vi "Modbus LDO Sensors.vi"(8 "error in":errorcluster, 11 "PLC Data":T1) -> (0 "error out":errorcluster, 3 "PLC Data Output":T1)   [LabVIEW 2020, in "Modbus.lvlib"]
uses:
  Modbus.lvlib
  Modbus PLC Data All.ctl
  Modbus FVIR Control.ctl
  Modbus LDO Control.ctl
  WritingDataFile/Data to Save.ctl
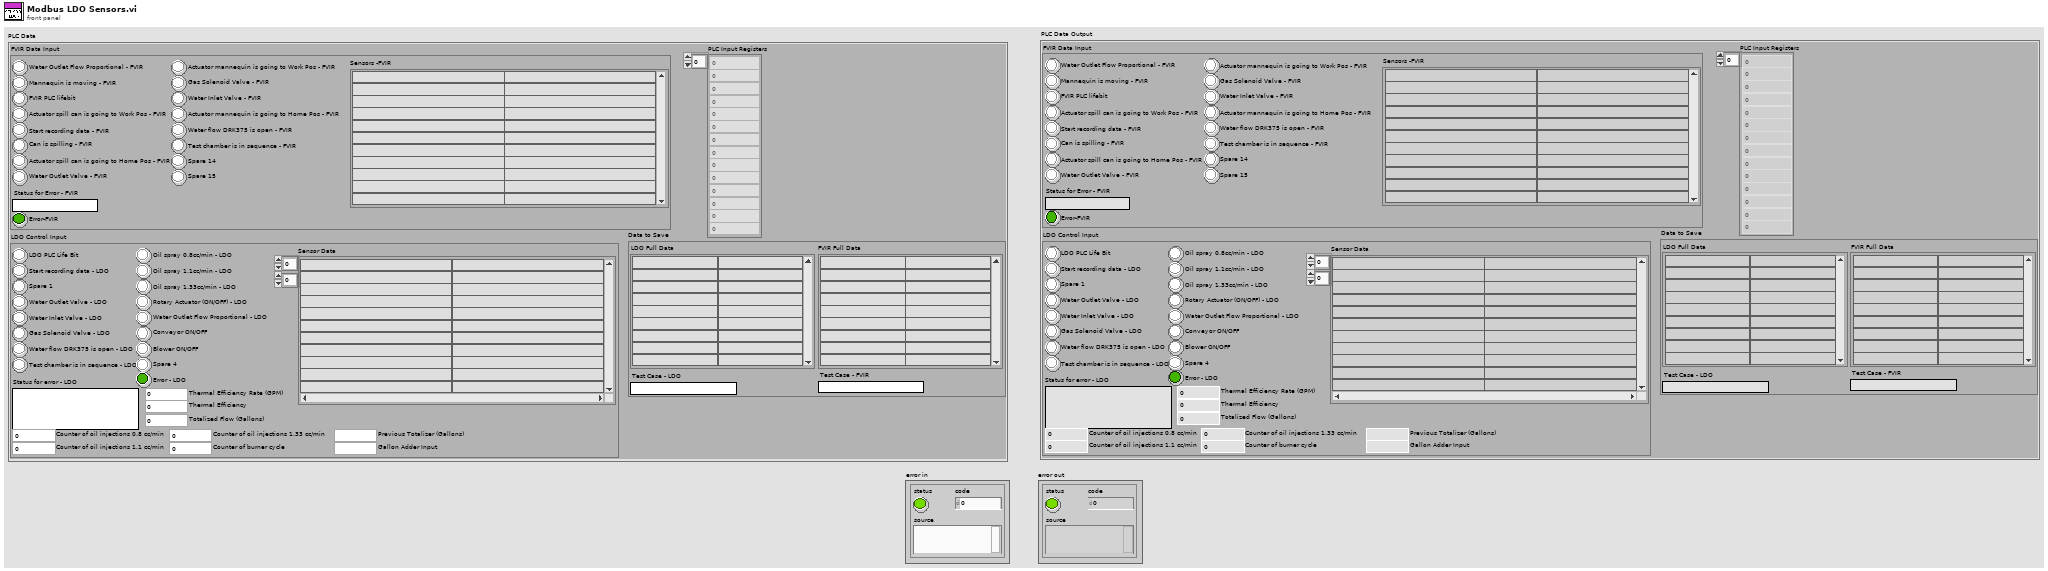
[diagram p1: front panel]
types:
  T1 = typedef "Modbus PLC Data All.ctl" = cluster{"FVIR Data Input":T2, "LDO Control Input":T3, "PLC Input Registers":i16[], "Data to Save":T4}
  T2 = typedef "Modbus FVIR Control.ctl" = cluster{"Spare 15":bool, "Spare 14":bool, "Actuator mannequin is going to Work Pos - FVIR":bool, "Actuator mannequin is going to Home Pos - FVIR":bool, "Test chamber is in sequence - FVIR ":bool, "Water flow DRK375 is open - FVIR":bool, "Gas Solenoid Valve - FVIR":bool, "Water Inlet Valve - FVIR":bool, "Water Outlet Flow Proportional - FVIR":bool, "Start recording data - FVIR":bool, "Actuator spill can is going to Work Pos - FVIR":bool, "Actuator spill can is going to Home Pos - FVIR":bool, "Water Outlet Valve - FVIR":bool, "Can is spilling - FVIR":bool, "Mannequin is moving - FVIR":bool, "FVIR PLC lifebit":bool, "Status for Error - FVIR":string, "Error-FVIR":bool, "Sensors -FVIR":string[][]}
  T3 = typedef "Modbus LDO Control.ctl" = cluster{"LDO PLC Life Bit":bool, "Start recording data - LDO":bool, "Spare 1":bool, "Water Outlet Valve - LDO":bool, "Water Inlet Valve - LDO":bool, "Gas Solenoid Valve - LDO":bool, "Water flow DRK375 is open - LDO":bool, "Test chamber is in sequence - LDO":bool, "Oil spray 0.8cc/min - LDO":bool, "Oil spray 1.1cc/min - LDO":bool, "Oil spray 1.33cc/min - LDO":bool, "Rotary Actuator (ON/OFF) - LDO":bool, "Water Outlet Flow Proportional - LDO":bool, "Conveyor ON/OFF":bool, "Blower ON/OFF":bool, "Spare 4":bool, "Status for error - LDO":string, "Error - LDO":bool, "Sensor Data":string[][], "Thermal Efficiency Rate (GPM)":dbl, "Thermal Efficiency":dbl, "Totalized Flow (Gallons)":dbl, "Counter of oil injections 1.33 cc/min":u16, "Counter of burner cycle":u16, "Counter of oil injections 1.1 cc/min":u16, "Counter of oil injections 0.8 cc/min":u16, "Previous Totalizer (Gallons)":dbl, "Gallon Adder Input":dbl}
  T4 = typedef "Data to Save.ctl" = cluster{"LDO Full Data":string[][], "FVIR Full Data":string[][], "Test Case - FVIR":string, "Test Case - LDO":string}
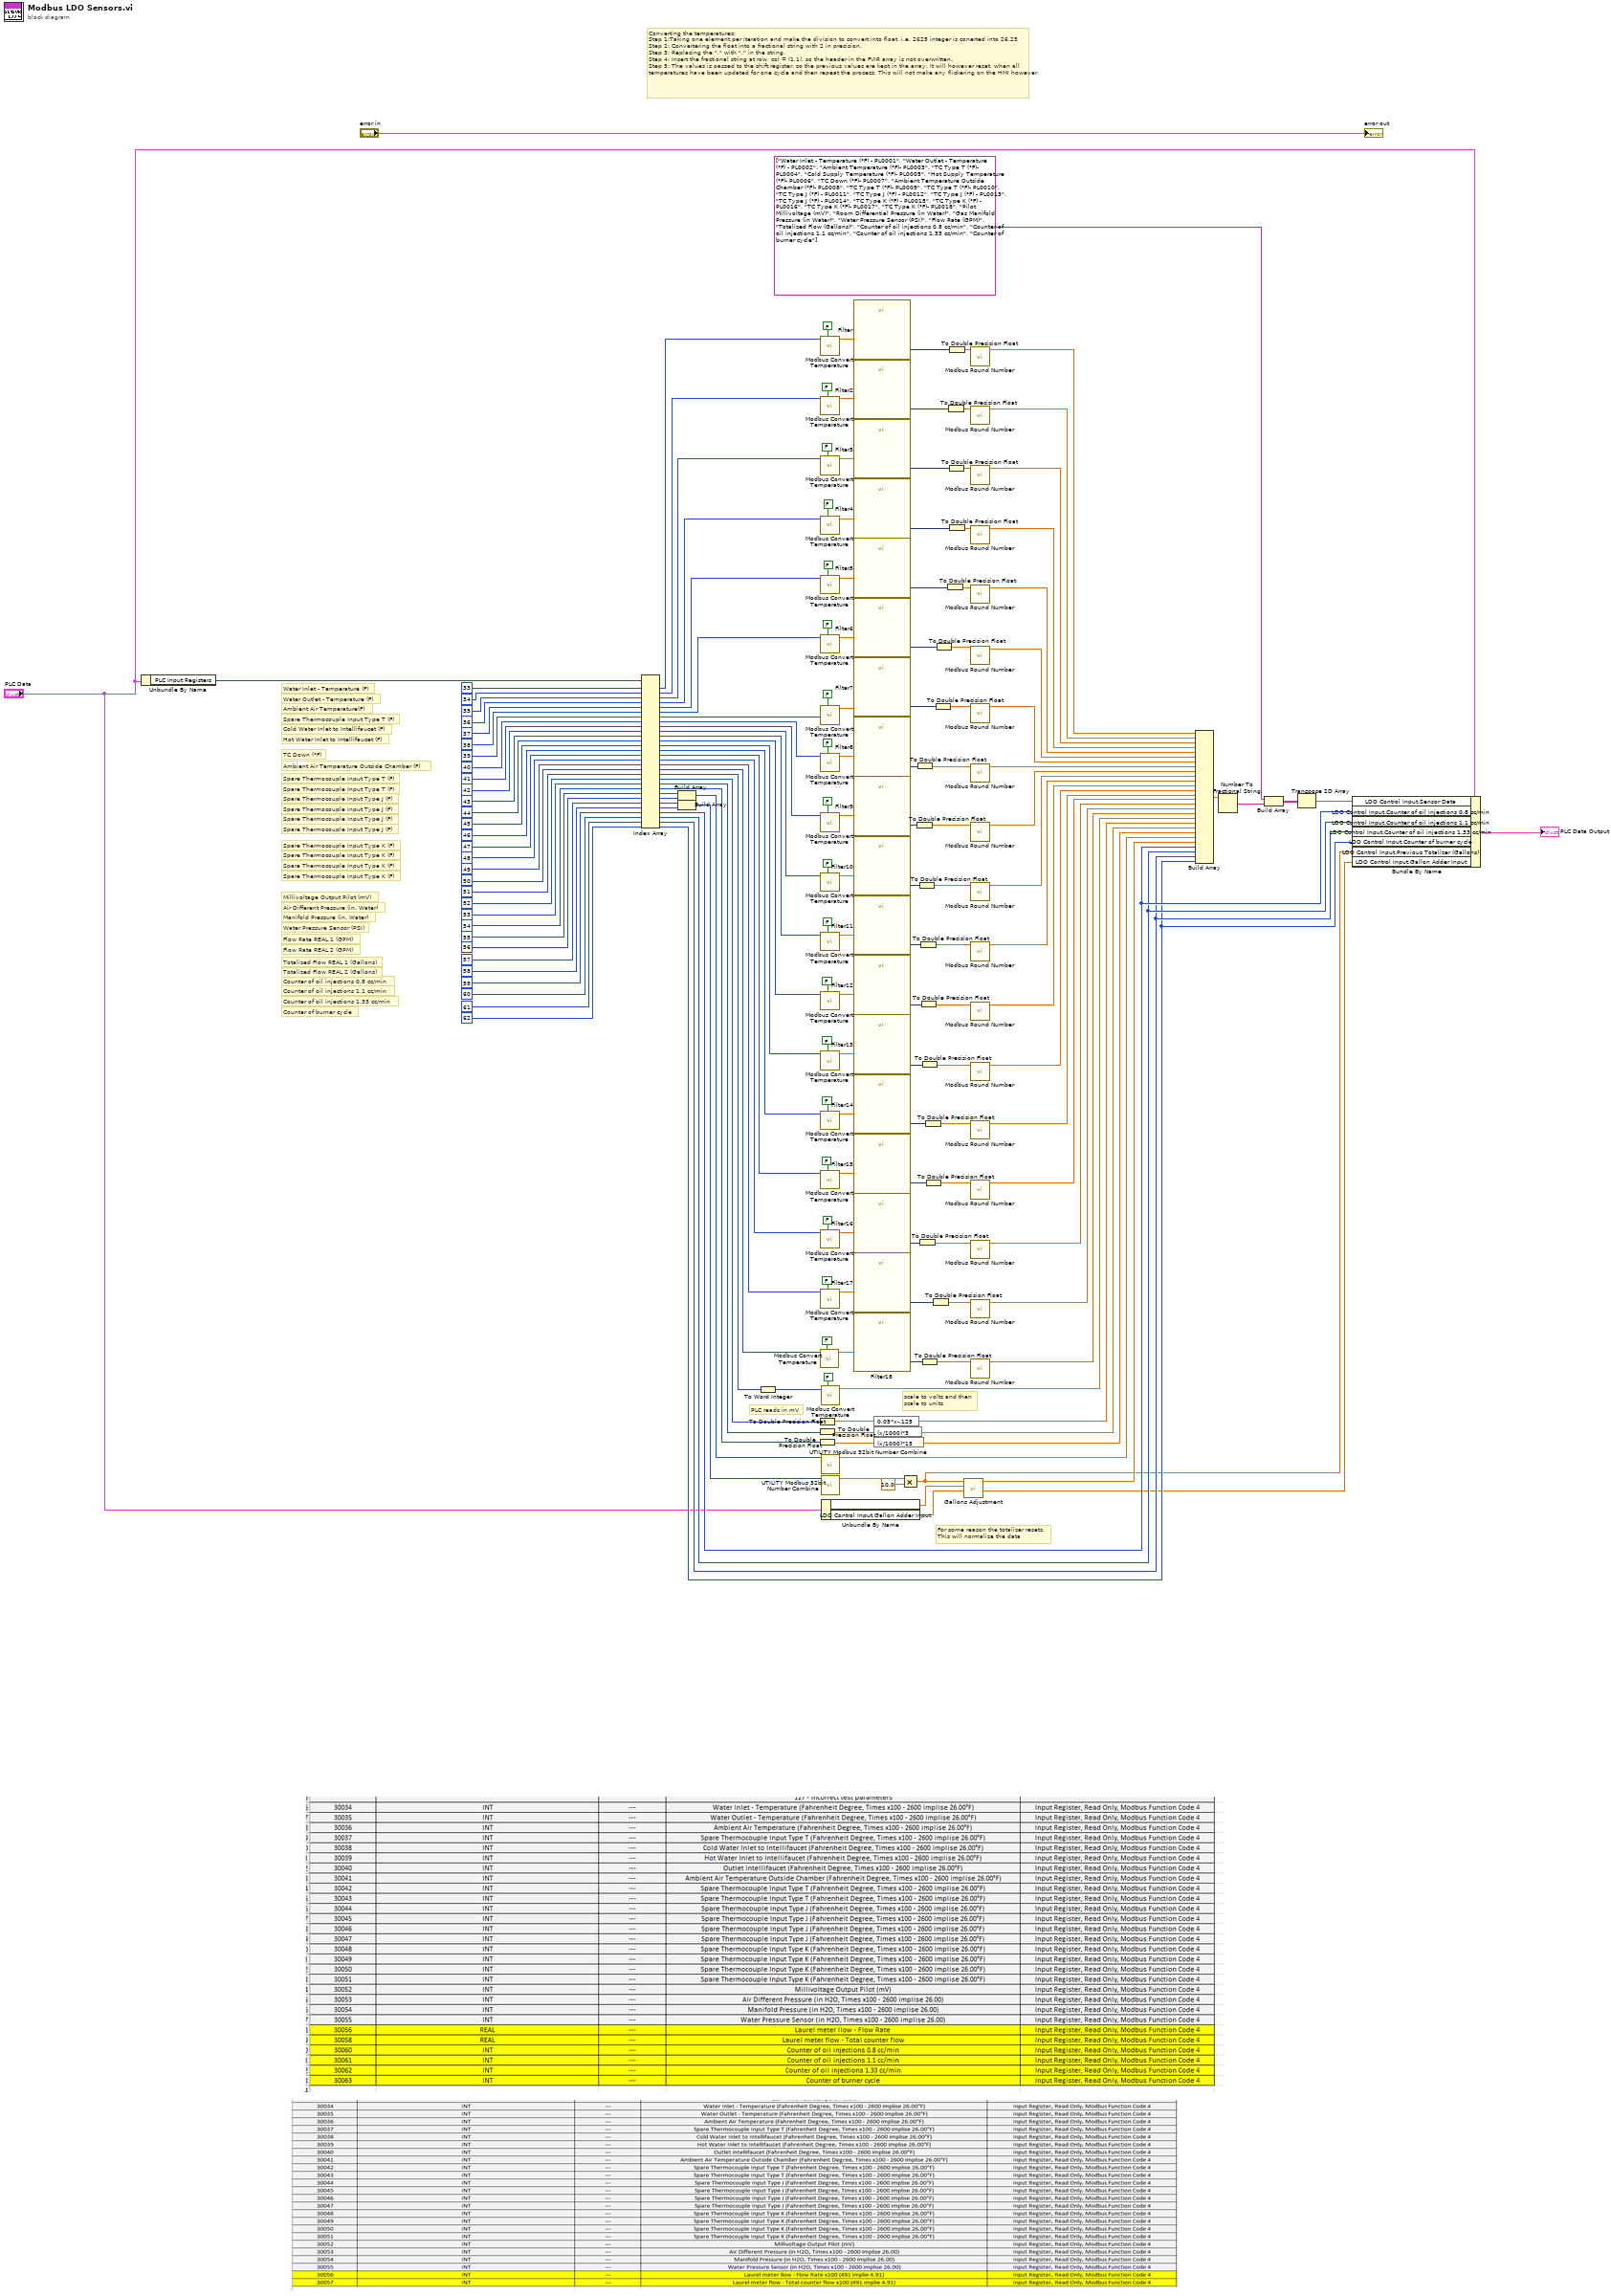
[diagram p0: block diagram]
diagram:
  # "For some reason the totalizer resets.\nThis will normalize the data"
  # "Counter of burner cycle"
  # "Counter of oil injections 1.33 cc/min"
  # "Counter of oil injections 1.1 cc/min"
  # "Counter of oil injections 0.8 cc/min"
  # "Totalized Flow REAL 2 (Gallons)"
  # "Totalized Flow REAL 1 (Gallons)"
  # "scale to volts and then \nscale to units"
  # "PLC reads in mV"
  # "Flow Rate REAL 2 (GPM)"
  # "Flow Rate REAL 1 (GPM)"
  # "Water Pressure Sensor (PSI)"
  # "Manifold Pressure (in. Water)"
  # "Air Different Pressure (in. Water)"
  # "Millivoltage Output Pilot (mV)"
  # "Spare Thermocouple Input Type K (F)"
  # "Spare Thermocouple Input Type K (F)"
  # "Spare Thermocouple Input Type K (F)"
  # "Spare Thermocouple Input Type K (F)"
  # "Spare Thermocouple Input Type J (F)"
  # "Spare Thermocouple Input Type J (F)"
  # "Spare Thermocouple Input Type J (F)"
  # "Spare Thermocouple Input Type J (F)"
  # "Spare Thermocouple Input Type T (F)"
  # "Spare Thermocouple Input Type T (F)"
  # "Ambient Air Temperature Outside Chamber (F)"
  # "TC Down (°F)"
  # "Hot Water Inlet to Intellifaucet (F)"
  # "Cold Water Inlet to Intellifaucet (F)"
  # "Spare Thermocouple Input Type T (F)"
  # "Ambient Air Temperature(F)"
  # "Water Outlet - Temperature (F)"
  # "Water Inlet - Temperature (F)"
  # "Converting the temperatures: \nStep 1:Taking one element per iteration and make the division to convert into float, i.e. 2625 integer is conerted into 26,25\nStep 2: Convertering the float into a fractional string with 2 in precision. \nStep 3: Replacing the \",\" with \".\" in the string.\nStep 4: Insert the fractional string at row, col = (1,1), so the header in the FVIR array is not overwritten. \nStep 5: The values is passed to the shift register, so the previous values are kept in the array. It will however reset, when all temperatures have been updated for one cycle and then repeat the process. This will not make any flickering on the HMI however."
  n1 = Unbundle By Name("PLC Data") -> ("PLC Input Registers"=w127:i16[])
  n2 = Index Array(array=w127, index #1=33 ("index"), index #2=34 ("index"), index #3=35 ("index"), index #4=36 ("index"), index #5=37 ("index"), index #6=38 ("index"), index #7=39 ("index"), index #8=40 ("index"), index #9=41 ("index"), index #10=42 ("index"), index #11=43 ("index"), index #12=44 ("index"), index #13=45 ("index"), index #14=46 ("index"), index #15=47 ("index"), index #16=48 ("index"), index #17=49 ("index"), index #18=50 ("index"), index #19=51 ("index"), index #20=52 ("index"), index #21=53 ("index"), index #22=54 ("index"), index #23=55 ("index"), index #24=56 ("index"), index #25=57 ("index"), index #26=58 ("index"), index #27=59 ("index"), index #28=60 ("index"), index #29=61 ("index"), index #30=62 ("index")) -> (element #1=w154:i16, element #2=w153:i16, element #3=w152:i16, element #4=w151:i16, element #5=w150:i16, element #6=w149:i16, element #7=w148:i16, element #8=w147:i16, element #9=w146:i16, element #10=w145:i16, element #11=w144:i16, element #12=w143:i16, element #13=w142:i16, element #14=w141:i16, element #15=w140:i16, element #16=w139:i16, element #17=w138:i16, element #18=w137:i16, element #19=w47:i16, element #20=w135:i16, element #21=w126:i16, element #22=w134:i16, element #23=w19:i16, element #24=w18:i16, element #25=w17:i16, element #26=w16:i16, element #27=w12:i16, element #28=w11:i16, element #29=w10:i16, element #30=w9:i16)
  n3 = Build Array(w19, w18) -> (w15:i16[])
  n4 = Build Array(w17, w16) -> (w14:i16[])
  n5 = To Word Integer(number=w47) -> (16bit integer=w27:i16)
  n6 = To Double Precision Float(number=w135) -> (double precision float=w124:dbl)
  n7 = To Double Precision Float(number=w126) -> (double precision float=w125:dbl)
  n8 = To Double Precision Float(number=w134) -> (double precision float=w121:dbl)
  n9 = call "Modbus Convert Temperature.vi"("Divide by 100?"=FALSE, "PLC Value"=w137) -> ("Converted Value"=w84:dbl)  [unwired: 8 in, 1 out]
  n10 = call "Modbus Convert Temperature.vi"("Divide by 100?"=FALSE, "PLC Value"=w154) -> ("Converted Value"=w119:dbl)  [unwired: 8 in, 1 out]
  n11 = call "Modbus Convert Temperature.vi"("Divide by 100?"=FALSE, "PLC Value"=w153) -> ("Converted Value"=w116:dbl)  [unwired: 8 in, 1 out]
  n12 = call "Modbus Convert Temperature.vi"("Divide by 100?"=FALSE, "PLC Value"=w152) -> ("Converted Value"=w114:dbl)  [unwired: 8 in, 1 out]
  n13 = call "Modbus Convert Temperature.vi"("Divide by 100?"=FALSE, "PLC Value"=w151) -> ("Converted Value"=w112:dbl)  [unwired: 8 in, 1 out]
  n14 = call "Modbus Convert Temperature.vi"("Divide by 100?"=FALSE, "PLC Value"=w150) -> ("Converted Value"=w110:dbl)  [unwired: 8 in, 1 out]
  n15 = call "Modbus Convert Temperature.vi"("Divide by 100?"=FALSE, "PLC Value"=w149) -> ("Converted Value"=w108:dbl)  [unwired: 8 in, 1 out]
  n16 = call "Modbus Convert Temperature.vi"("Divide by 100?"=FALSE, "PLC Value"=w148) -> ("Converted Value"=w106:dbl)  [unwired: 8 in, 1 out]
  n17 = call "Modbus Convert Temperature.vi"("Divide by 100?"=FALSE, "PLC Value"=w147) -> ("Converted Value"=w104:dbl)  [unwired: 8 in, 1 out]
  n18 = call "Modbus Convert Temperature.vi"("Divide by 100?"=FALSE, "PLC Value"=w146) -> ("Converted Value"=w102:dbl)  [unwired: 8 in, 1 out]
  n19 = call "Modbus Convert Temperature.vi"("Divide by 100?"=FALSE, "PLC Value"=w145) -> ("Converted Value"=w100:dbl)  [unwired: 8 in, 1 out]
  n20 = call "Modbus Convert Temperature.vi"("Divide by 100?"=FALSE, "PLC Value"=w144) -> ("Converted Value"=w98:dbl)  [unwired: 8 in, 1 out]
  n21 = call "Modbus Convert Temperature.vi"("Divide by 100?"=FALSE, "PLC Value"=w143) -> ("Converted Value"=w96:dbl)  [unwired: 8 in, 1 out]
  n22 = call "Modbus Convert Temperature.vi"("Divide by 100?"=FALSE, "PLC Value"=w142) -> ("Converted Value"=w94:dbl)  [unwired: 8 in, 1 out]
  n23 = call "Modbus Convert Temperature.vi"("Divide by 100?"=FALSE, "PLC Value"=w141) -> ("Converted Value"=w92:dbl)  [unwired: 8 in, 1 out]
  n24 = call "Modbus Convert Temperature.vi"("Divide by 100?"=FALSE, "PLC Value"=w140) -> ("Converted Value"=w90:dbl)  [unwired: 8 in, 1 out]
  n25 = call "Modbus Convert Temperature.vi"("Divide by 100?"=FALSE, "PLC Value"=w139) -> ("Converted Value"=w88:dbl)  [unwired: 8 in, 1 out]
  n26 = call "Modbus Convert Temperature.vi"("Divide by 100?"=FALSE, "PLC Value"=w138) -> ("Converted Value"=w86:dbl)  [unwired: 8 in, 1 out]
  n27 = call "Modbus Convert Temperature.vi"("Divide by 100?"=FALSE, "PLC Value"=w27) -> ("Converted Value"=w26:dbl)  [unwired: 8 in, 1 out]
  n28 = call "UTILITY Modbus 32bit Number Combine.vi"("Holding Registers"=w15) -> ("Data"=w13:sgl)  [unwired: 9 in, 1 out]
  n29 = call "UTILITY Modbus 32bit Number Combine.vi"("Holding Registers"=w14) -> ("Data"=w8:sgl)  [unwired: 9 in, 1 out]
  n30 = Unbundle By Name("PLC Data") -> ("LDO Control Input.Previous Totalizer (Gallons)"=w5:dbl, "LDO Control Input.Gallon Adder Input"=w4:dbl)
  n31 = call "Filter"("Signal"=w119) -> ("Filtered Signal"=w118:dynamicdata)  [unwired: 9 in, 1 out]
  n32 = call "Filter2"("Signal"=w116) -> ("Filtered Signal"=w117:dynamicdata)  [unwired: 9 in, 1 out]
  n33 = call "Filter3"("Signal"=w114) -> ("Filtered Signal"=w115:dynamicdata)  [unwired: 9 in, 1 out]
  n34 = call "Filter4"("Signal"=w112) -> ("Filtered Signal"=w113:dynamicdata)  [unwired: 9 in, 1 out]
  n35 = call "Filter5"("Signal"=w110) -> ("Filtered Signal"=w111:dynamicdata)  [unwired: 9 in, 1 out]
  n36 = call "Filter6"("Signal"=w108) -> ("Filtered Signal"=w109:dynamicdata)  [unwired: 9 in, 1 out]
  n37 = call "Filter7"("Signal"=w106) -> ("Filtered Signal"=w107:dynamicdata)  [unwired: 9 in, 1 out]
  n38 = call "Filter8"("Signal"=w104) -> ("Filtered Signal"=w105:dynamicdata)  [unwired: 9 in, 1 out]
  n39 = call "Filter9"("Signal"=w102) -> ("Filtered Signal"=w103:dynamicdata)  [unwired: 9 in, 1 out]
  n40 = call "Filter10"("Signal"=w100) -> ("Filtered Signal"=w101:dynamicdata)  [unwired: 9 in, 1 out]
  n41 = call "Filter11"("Signal"=w98) -> ("Filtered Signal"=w99:dynamicdata)  [unwired: 9 in, 1 out]
  n42 = call "Filter12"("Signal"=w96) -> ("Filtered Signal"=w97:dynamicdata)  [unwired: 9 in, 1 out]
  n43 = call "Filter13"("Signal"=w94) -> ("Filtered Signal"=w95:dynamicdata)  [unwired: 9 in, 1 out]
  n44 = call "Filter14"("Signal"=w92) -> ("Filtered Signal"=w93:dynamicdata)  [unwired: 9 in, 1 out]
  n45 = call "Filter15"("Signal"=w90) -> ("Filtered Signal"=w91:dynamicdata)  [unwired: 9 in, 1 out]
  n46 = call "Filter16"("Signal"=w88) -> ("Filtered Signal"=w89:dynamicdata)  [unwired: 9 in, 1 out]
  n47 = call "Filter17"("Signal"=w86) -> ("Filtered Signal"=w87:dynamicdata)  [unwired: 9 in, 1 out]
  n48 = call "Filter18"("Signal"=w84) -> ("Filtered Signal"=w85:dynamicdata)  [unwired: 9 in, 1 out]
  n49 = expression code="0.05*x-.125"(w124) -> (w123:dbl)
  n50 = expression code="(x/1000)*3"(w125) -> (w122:dbl)
  n51 = expression code="(x/1000)*15"(w121) -> (w120:dbl)
  n52 = Multiply(x=w8, y=sgl 10.0) -> (x*y=w1:sgl)
  n53 = To Double Precision Float(number=w103) -> (double precision float=w67:dbl)
  n54 = To Double Precision Float(number=w105) -> (double precision float=w69:dbl)
  n55 = To Double Precision Float(number=w101) -> (double precision float=w65:dbl)
  n56 = To Double Precision Float(number=w89) -> (double precision float=w53:dbl)
  n57 = To Double Precision Float(number=w99) -> (double precision float=w63:dbl)
  n58 = To Double Precision Float(number=w97) -> (double precision float=w61:dbl)
  n59 = To Double Precision Float(number=w95) -> (double precision float=w59:dbl)
  n60 = To Double Precision Float(number=w85) -> (double precision float=w49:dbl)
  n61 = To Double Precision Float(number=w93) -> (double precision float=w57:dbl)
  n62 = To Double Precision Float(number=w91) -> (double precision float=w55:dbl)
  n63 = To Double Precision Float(number=w87) -> (double precision float=w51:dbl)
  n64 = To Double Precision Float(number=w107) -> (double precision float=w71:dbl)
  n65 = To Double Precision Float(number=w109) -> (double precision float=w73:dbl)
  n66 = To Double Precision Float(number=w111) -> (double precision float=w75:dbl)
  n67 = To Double Precision Float(number=w117) -> (double precision float=w81:dbl)
  n68 = To Double Precision Float(number=w115) -> (double precision float=w79:dbl)
  n69 = To Double Precision Float(number=w118) -> (double precision float=w83:dbl)
  n70 = To Double Precision Float(number=w113) -> (double precision float=w77:dbl)
  n71 = call "Gallons Adjustment.vi"("Gallon Adder Input"=w4, "Previous Totalizer (Gallons)"=w5, "Current Totalizer (Gallons)"=w1) -> ("Gallon Adder Output"=w2:dbl, "Normalized Gallons"=w3:dbl)  [unwired: 7 in]
  n72 = call "Modbus Round Number.vi"("Number"=w83) -> ("Rounded Number"=w82:dbl)  [unwired: 10 in]
  n73 = call "Modbus Round Number.vi"("Number"=w81) -> ("Rounded Number"=w80:dbl)  [unwired: 10 in]
  n74 = call "Modbus Round Number.vi"("Number"=w79) -> ("Rounded Number"=w78:dbl)  [unwired: 10 in]
  n75 = call "Modbus Round Number.vi"("Number"=w77) -> ("Rounded Number"=w76:dbl)  [unwired: 10 in]
  n76 = call "Modbus Round Number.vi"("Number"=w75) -> ("Rounded Number"=w74:dbl)  [unwired: 10 in]
  n77 = call "Modbus Round Number.vi"("Number"=w73) -> ("Rounded Number"=w72:dbl)  [unwired: 10 in]
  n78 = call "Modbus Round Number.vi"("Number"=w71) -> ("Rounded Number"=w70:dbl)  [unwired: 10 in]
  n79 = call "Modbus Round Number.vi"("Number"=w69) -> ("Rounded Number"=w68:dbl)  [unwired: 10 in]
  n80 = call "Modbus Round Number.vi"("Number"=w67) -> ("Rounded Number"=w66:dbl)  [unwired: 10 in]
  n81 = call "Modbus Round Number.vi"("Number"=w65) -> ("Rounded Number"=w64:dbl)  [unwired: 10 in]
  n82 = call "Modbus Round Number.vi"("Number"=w63) -> ("Rounded Number"=w62:dbl)  [unwired: 10 in]
  n83 = call "Modbus Round Number.vi"("Number"=w61) -> ("Rounded Number"=w60:dbl)  [unwired: 10 in]
  n84 = call "Modbus Round Number.vi"("Number"=w59) -> ("Rounded Number"=w58:dbl)  [unwired: 10 in]
  n85 = call "Modbus Round Number.vi"("Number"=w57) -> ("Rounded Number"=w56:dbl)  [unwired: 10 in]
  n86 = call "Modbus Round Number.vi"("Number"=w55) -> ("Rounded Number"=w54:dbl)  [unwired: 10 in]
  n87 = call "Modbus Round Number.vi"("Number"=w53) -> ("Rounded Number"=w52:dbl)  [unwired: 10 in]
  n88 = call "Modbus Round Number.vi"("Number"=w51) -> ("Rounded Number"=w50:dbl)  [unwired: 10 in]
  n89 = call "Modbus Round Number.vi"("Number"=w49) -> ("Rounded Number"=w48:dbl)  [unwired: 10 in]
  n90 = Build Array(w82, w80, w78, w76, w74, w72, w70, w68, w66, w64, w62, w60, w58, w56, w54, w52, w50, w48, w26, w123, w122, w120, w13, w3, w12, w11, w10, w9) -> (w133:dbl[])
  n91 = Number To Fractional String(number=w133) -> (F-format string=w132:string[])  [unwired: 3 in]
  n92 = Build Array(string[] ["Water Inlet - Temperature (°F) - PL0001", "Water Outlet - Temperature (°F) - PL0002", "Ambient Temperature (°F)- PL0003", "TC Type T (°F)- PL0004", "Cold Supply Temperature (°F)- PL0005", "Hot Supply Temperature (°F)- PL0006", "TC Down (°F)- PL0007", "Ambient Temperature Outside Chamber (°F)- PL0008", "TC Type T (°F)- PL0009", "TC Type T (°F)- PL0010", "TC Type J (°F) - PL0011", "TC Type J (°F) - PL0012", "TC Type J (°F) - PL0013", "TC Type J (°F) - PL0014", "TC Type K (°F) - PL0015", "TC Type K (°F) - PL0016", "TC Type K (°F)- PL0017", "TC Type K (°F)- PL0018", "Pilot Millivoltage (mV)", "Room Differential Pressure (in Water)", "Gas Manifold Pressure (in Water)", "Water Pressure Sensor (PSI)", "Flow Rate (GPM)", "Totalized Flow (Gallons)", "Counter of oil injections 0.8 cc/min", "Counter of oil injections 1.1 cc/min", "Counter of oil injections 1.33 cc/min", "Counter of burner cycle"] ("Array 2"), w132) -> (w130:string[][])
  n93 = Transpose 2D Array(2D array=w130) -> (transposed array=w129:string[][])
  n94 = Bundle By Name(cluster="PLC Data", "LDO Control Input.Sensor Data"=w129, "LDO Control Input.Counter of oil injections 0.8 cc/min"=w12, "LDO Control Input.Counter of oil injections 1.1 cc/min"=w11, "LDO Control Input.Counter of oil injections 1.33 cc/min"=w10, "LDO Control Input.Counter of burner cycle"=w9, "LDO Control Input.Previous Totalizer (Gallons)"=w1, "LDO Control Input.Gallon Adder Input"=w2) -> (→"PLC Data Output":T1)
  "error out" <- "error in"
